vi "Make Size String.vi"(8 "error in (no error)":errorcluster, 9 "Height (480)":u16=480 min=1 max=640, 10 "Width (480)":u16=480 min=1 max=640) -> (0 "error out":errorcluster, 2 "Size string":string)   [LabVIEW 2012]
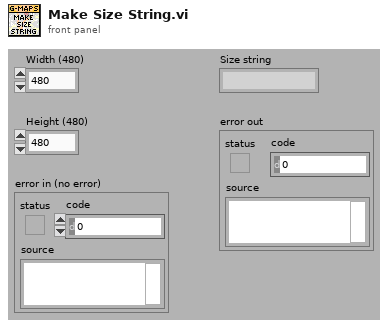
[diagram p1: front panel]
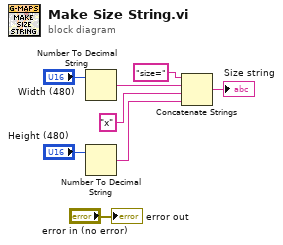
[diagram p0: block diagram]
diagram:
  n1 = Number To Decimal String(number="Width (480)") -> (decimal integer string=w1:string)  [unwired: 1 in]
  n2 = Number To Decimal String(number="Height (480)") -> (decimal integer string=w3:string)  [unwired: 1 in]
  n3 = Concatenate Strings("size=" ("URL"), w1, "x" ("URL"), w3) -> (→"Size string":string)
  "error out" <- "error in (no error)"
